vi "calc_fid_transform.vi"(3 "PairedFiducialCoordinates":T3[](array[typedef])) -> (2 "error":i32 format="%.3p", 4 "Transformation_Matrices":T2, 5 "FidcucialMetrics":cluster{"M1":dbl, "M2":dbl, "S1":dbl, "S2":dbl}, 6 "Matrices_in_text":string, 7 "ShiftedPairedFiducials":T3)   [LabVIEW 2011]
doc: "This VI sets up and calls the routines to calculate the tranformation matrix and vectors to tranform a point in the reference session to the current session coordinate system.\n\nA(x-c) + b = y\nWhere x is a coordinate in the reference session,\ny is the transformation of that coordinate into the current session.\nc is the translation of the reference point to that of the common point of rotation\nb is the translation of the current session coordinates to the common point of rotation\nA is the rotation and scaling matrix for the transformation.\n\nThe first paired set of fiducials from the list is used as the common point of rotation. The location of the first reference session fiducials is \"c\"\n\nAll fiducials are translated by the negative of the first paired fiducial to enable the calculation of A. \n\nThe PairedFiducial locations, c, and A are used to find B as the mean of the displacement of the rotated and scaled fiducials from there known locations in the current session coordinate system. This should be approximately the location of the first fiducial in the current session coordinate system."
uses:
  Fiducial_pair.ctl
  transformMatrix.ctl
  <vilib>/Analysis/Matrix/Datatypes/RealMatrix.ctl
  <vilib>/Analysis/Matrix/Numeric/Conversions/Array To Matrix - RA.vi
  <vilib>/Analysis/Matrix/Numeric/Conversions/Matrix To Array - RM.vi
  <vilib>/Analysis/Matrix/NI_Matrix.lvlib
panel:
  out "pinv(X')":T1
  out "X'":T1
  out "Y'":T1
  # "Fiducial Location Pair"
  # "Current Instrument Fiducial Location"
  # "Reference Instrument Fiducial Location"
  # "Fiducial Location Pair"
  # "Current Instrument Fiducial Location"
  # "Reference Instrument Fiducial Location"
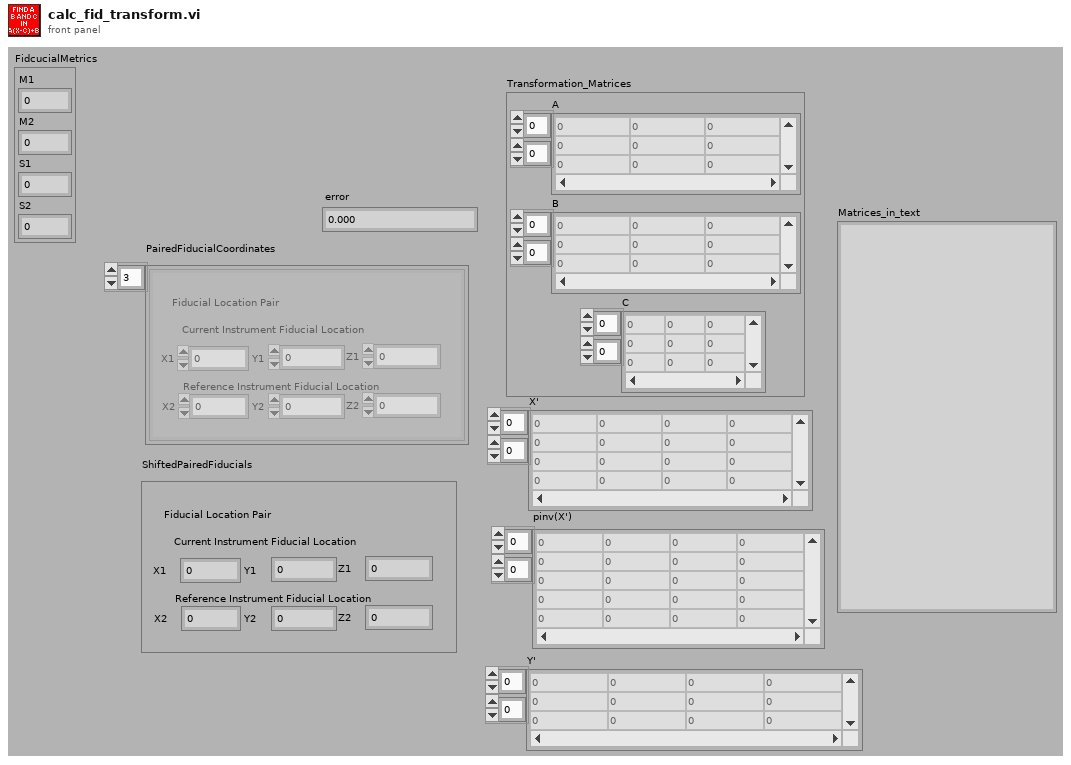
[diagram p1: front panel]
types:
  T1 = typedef "NI_Matrix.lvlib/RealMatrix.ctl" = dbl[][]
  T2 = typedef "transformMatrix.ctl" = cluster{"A":T1, "B":T1, "C":T1}
  T3 = typedef "Fiducial_pair.ctl" = cluster{"X1":dbl, "X2":dbl, "Y1":dbl, "Y2":dbl, "Z1":dbl, "Z2":dbl}
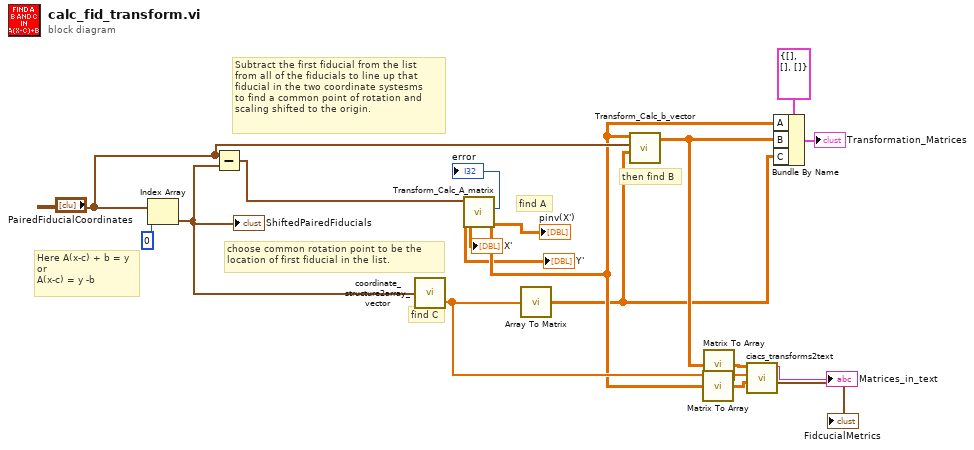
[diagram p0: block diagram]
diagram:
  # "then find B"
  # "find A"
  # "find C"
  # "choose common rotation point to be the\nlocation of first fiducial in the list."
  # "Subtract the first fiducial from the list\nfrom all of the fiducials to line up that\nfiducial in the two coordinate systesms\nto find a common point of rotation and\nscaling shifted to the origin."
  # "Here A(x-c) + b = y\nor\nA(x-c) = y -b"
  n1 = Index Array(array="PairedFiducialCoordinates", index=0) -> (element=w17:T3)
  "ShiftedPairedFiducials" <- w17
  n2 = Subtract(x="PairedFiducialCoordinates", y=w17) -> (x-y=w16:T3[])
  n3 = call "coordinate_structure2array_vector.vi"("Fiducial_Pos_structure"=w17) -> ("Reference_Instrument_pos"=w13:dbl[])  [unwired: 1 out]
  n4 = call "Transform_Calc_A_matrix.vi"("PairedFiducialCoordinates"=w16) -> ("pinv(X')"=→"pinv(X')":T1, "A"=w8:T1, "error"=→"error":i32, "X'"=→"X'":T1, "Y'"=→"Y'":T1)  [unwired: 6 in]
  n5 = call-poly <vilib>:"Array To Matrix.vi"("Real 1D Array"=w13) -> ("Real Matrix (Column Vector)"=w6:T1)
  n6 = call "Transform_Calc_b_vector.vi"("C"=w6, "PairedFiducialCoordinates"="PairedFiducialCoordinates", "A"=w8) -> ("b"=w7:T1)  [unwired: 8 in]
  n7 = call-poly <vilib>:"Matrix To Array.vi"("Real Matrix"=w8) -> ("Real 2D Array"=w2:dbl[][])
  n8 = call-poly <vilib>:"Matrix To Array.vi"("Real Matrix"=w7) -> ("Real 2D Array"=w12:dbl[][])
  n9 = call "ciacs_transforms2text.vi"("A_transform"=w2, "C"=w13, "B"=w12) -> ("FidcucialMetrics"=→"FidcucialMetrics":cluster{"M1":dbl, "M2":dbl, "S1":dbl, "S2":dbl}, "Text of Transformation"=→"Matrices_in_text":string)  [unwired: 7 in]
  n10 = Bundle By Name(cluster=T2 {"A"=[], "B"=[], "C"=[]} ("Transformation_Matrices 2"), "A"=w8, "B"=w7, "C"=w6) -> (→"Transformation_Matrices":T2)
